vi "mouseRead.vi"() -> ()   [LabVIEW 2010]
panel:
  out "Cycles \ncompleted":dbl format="%#_2g"
  in  "DPI":dbl=350.0
  in  "Boolean":bool
  out "Numeric 3":dbl
  out "Numeric 2":dbl
  out "Numeric":dbl
  out "Waveform Chart":dbl(graph)
  out "Waveform Graph":dynamicdata(graph)
  in  "stop":bool
  in  "VISA Resource Name":refnum<visa-resource-name>
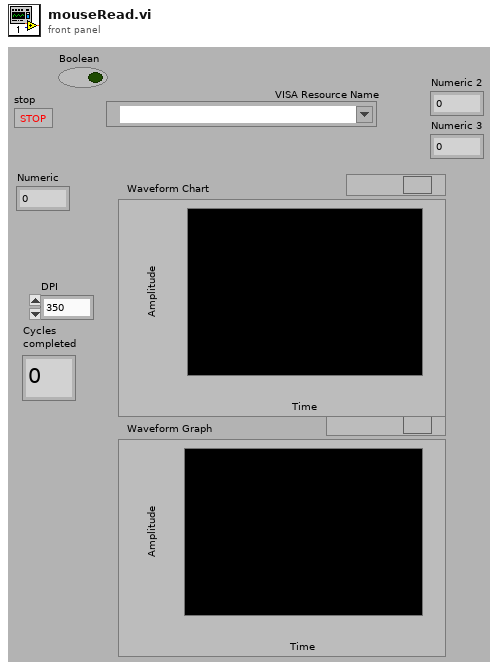
[diagram p1: front panel]
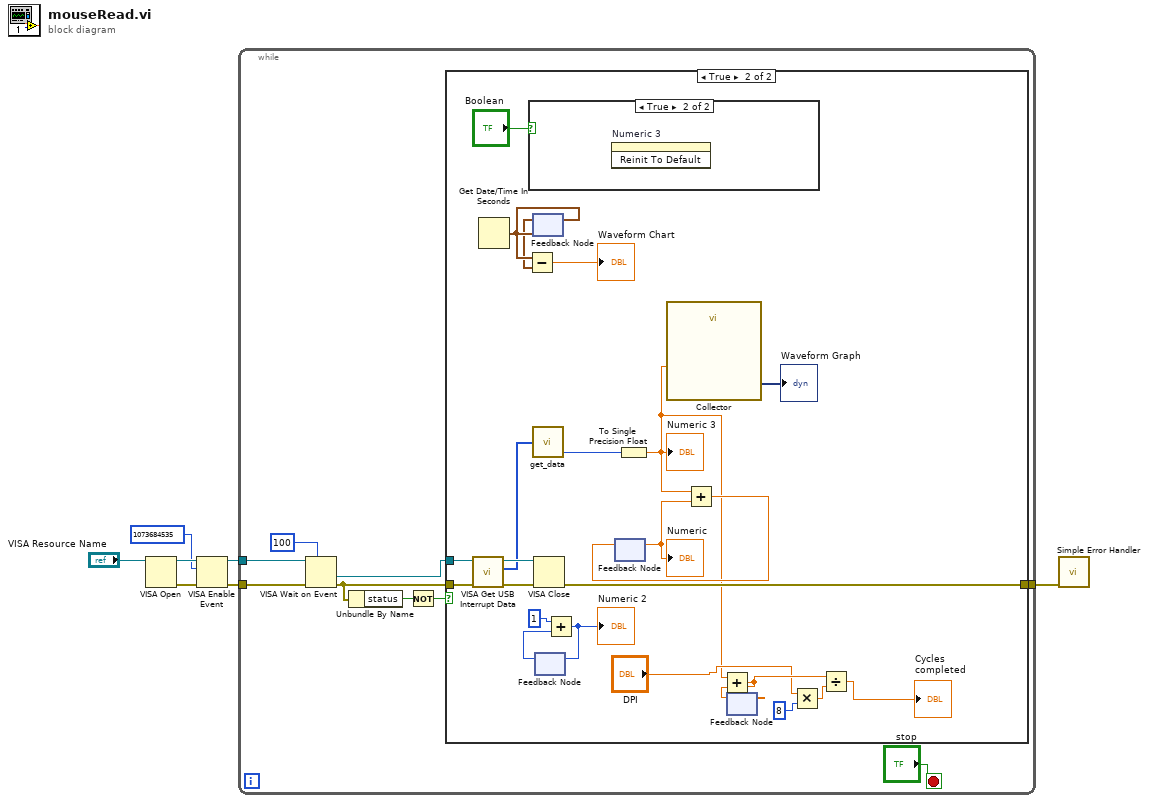
[diagram p0: block diagram]
diagram:
  n1 = VISA Open(VISA resource name="VISA Resource Name") -> (VISA resource name=w7:refnum<visa-resource-name>, error out=w6:errorcluster)  [unwired: 1 in, 3 out]
  n2 = VISA Enable Event(8:w6, 10:u32 1073684535 ("event type"), 11:w7) -> (0:w3:errorcluster, 3:w4:refnum<visa-resource-name>)  [unwired: 1 out]
  n3 = while {
    tunnel: w4 -> [w16]
    tunnel: w3 -> [w15]
    tunnel: [w9] -> w1
    stop <- "stop" stop-if-true
    n4 = VISA Wait on Event(7:u32 100 ("timeout (0)"), 8:w15, 11:w16) -> (0:w8:errorcluster, 1:w10:refnum<visa-resource-name>)  [unwired: 4 out]
    n5 = Unbundle By Name(w8) -> ("status"=w11:bool)
    n6 = Not(x=w11) -> (.not. x?=w12:bool)
    n7 = case shown="True" w12 {
      tunnel: w10 -> [_ w35]
      tunnel: [w17 w34] -> w9
      tunnel: w8 -> [w17 w33]
      frame False {
      }
      frame True {
        n8 = call <vilib>:"VISA Get USB Interrupt Data.vi"("error in (no error)"=w33, "VISA USB Intr Event"=w35) -> ("error out"=w36:errorcluster, "data buffer"=w32:u8[], "VISA USB Intr Event out"=w37:refnum<visa-resource-name>)  [unwired: 7 out]
        n9 = Get Date/Time In Seconds() -> (seconds since 1Jan1904=w40:timestamp)
        n10 = case shown="True" "Boolean" {
          frame False {
          }
          frame True {
            n11 = invoke on="Numeric 3" class="DigNum (strict)" method="Reinit To Default"() -> ()  [unwired: 3 in, 3 out]
          }
        }
        n12 = feedback #1(w40) -> (w39:timestamp)
        n13 = Subtract(x=w40, y=w39) -> (x-y=→"Waveform Chart":dbl)
        n14 = feedback-in #1(w40) -> ()
        n15 = call "get_data.vi"("data buffer"=w32) -> ("Y Value"=w26:i8)  [unwired: 2 out]
        n16 = VISA Close(VISA resource name=w37, error in (no error)=w36) -> (error out=w34:errorcluster)
        n17 = feedback #2() -> (w30:i32)  [unwired: 1 in]
        n18 = Add(x=1, y=w30) -> (x+y=w29:i32)
        "Numeric 2" <- w29
        n19 = feedback-in #2(w29) -> ()
        n20 = feedback #3() -> (w27:sgl)  [unwired: 1 in]
        "Numeric" <- w27
        n21 = To Single Precision Float(number=w26) -> (single precision float=w19:sgl)
        "Numeric 3" <- w19
        n22 = call "Collector"("Signals"=w19) -> ("Collected Signals"=→"Waveform Graph":dynamicdata)  [unwired: 9 in, 1 out]
        n23 = Add(x=w19, y=w27) -> (x+y=w28:sgl)
        n24 = feedback-in #3(w28) -> ()
        n25 = feedback #4() -> (w24:sgl)  [unwired: 1 in]
        n26 = Add(x=w19, y=w24) -> (x+y=w22:sgl)
        n27 = feedback-in #4(w22) -> ()
        n28 = Multiply(x="DPI", y=8) -> (x*y=w23:dbl)
        n29 = Divide(x=w22, y=w23) -> (x/y=→"Cycles \ncompleted":dbl)
      }
    }
  }
  n30 = call <vilib>:"Simple Error Handler.vi"("error in (no error)"=w1) -> ()  [unwired: 1 in, 8 out]
